vi "Sgl_to_Half_Prec_Array.vi"(5 "SGL":sgl[](array[numeric])) -> (2 "Half":u16[](array[numeric]) format="%016b")   [LabVIEW 2015]
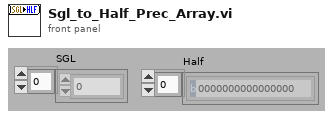
[diagram p1: front panel]
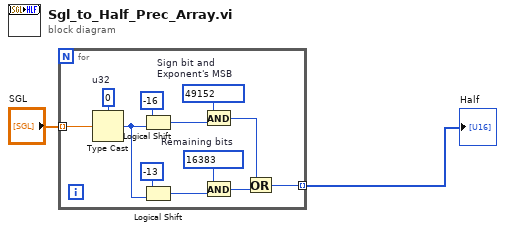
[diagram p0: block diagram]
diagram:
  n1 = for {
    tunnel: "SGL" -> [w4] mode=indexing
    tunnel: [w3] -> w1 mode=indexing
    w8 = u32 0  # u32
    w11 = u32 16383  # Remaining bits
    w14 = u32 49152  # Sign bit and Exponent's MSB
    n2 = Type Cast(type=w8, x=w4) -> (*(type *) &x=w6:u32)
    n3 = Logical Shift(y=-16, x=w6) -> (x << y=w5:u32)
    n4 = Logical Shift(y=-13, x=w6) -> (x << y=w12:u32)
    n5 = And(x=w14, y=w5) -> (x .and. y?=w9:u32)
    n6 = And(x=w11, y=w12) -> (x .and. y?=w10:u32)
    n7 = Or(x=w9, y=w10) -> (x .or. y?=w3:u32)
  }
  "Half" <- w1
